vi "仪器电源管理.vi"() -> ()   [LabVIEW 2016, in "环境动力监测库.lvlib" / "电源管理库.lvlib"]
uses:
  <vilib>/Utility/miscctls.llb/LVPointTypeDef.ctl
panel:
  out "R115":i16 caption="灯带关闭时间"
  out "R114":i16 caption="灯带开启时间"
  in  "视频监控":bool
  in  "照明":bool
  in  "前门灯带":bool
  in  "侧边灯带":bool
  in  "电源控制":T1
  in  "副屏看门狗启用":u16(ring) caption="副屏看门狗启用：" items=["关闭", "打开"]
  in  "副屏看门狗设置":u16 caption="副屏看门狗设置："
  out "副屏看门狗计时":u16 caption="副屏看门狗计时："
  in  "主屏看门狗启用":u16(ring) caption="主屏看门狗启用：" items=["关闭", "打开"]
  in  "主屏看门狗设置":u16 caption="主屏看门狗设置："
  out "主屏看门狗计时":u16 caption="主屏看门狗计时："
  # "仪器电源管理"
  # "s"
  # "s"
  # "s"
  # "s"
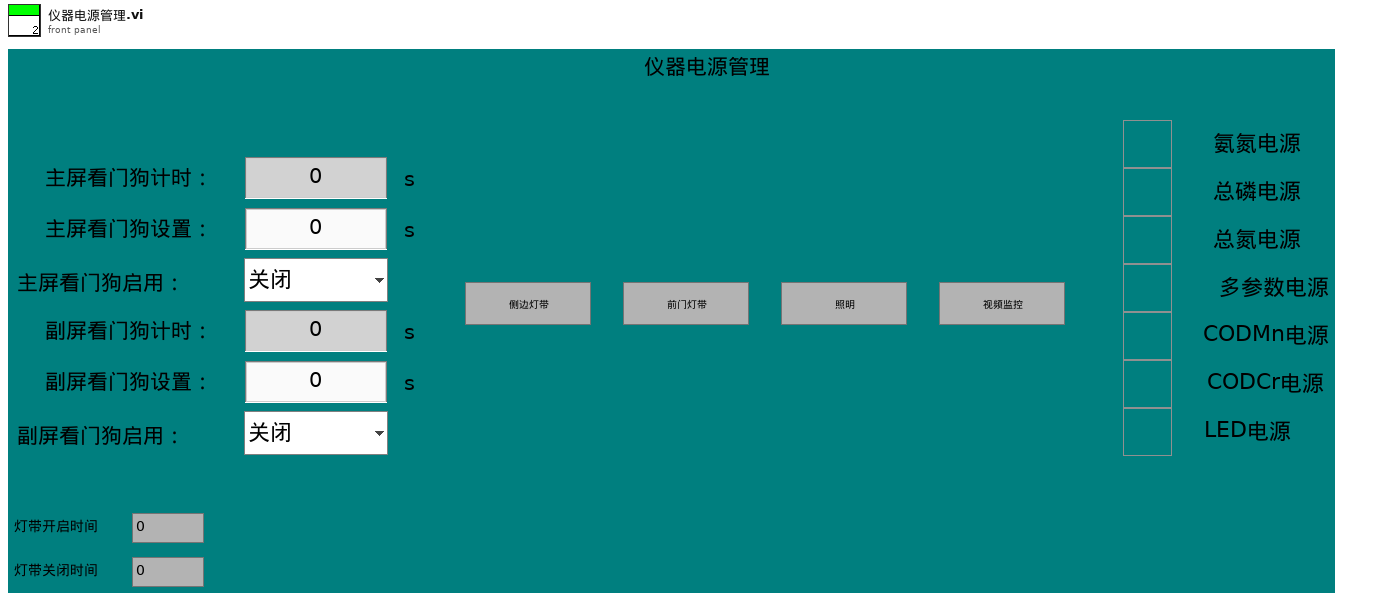
[diagram p1: front panel]
types:
  T1 = cluster{"氨氮电源":bool, "总磷电源":bool, "总氮电源":bool, "多参数电源":bool, "CODMn电源":bool, "CODCr电源":bool, "LED电源":bool}
  T2 = typedef "LVPointTypeDef.ctl" = cluster{"Horizontal":i16, "Vertical":i16}
  T3 = cluster{"R0":i16, "R1":i16, "R2":i16, "R3":i16, "R4":i16, "R5":i16, "R6":i16, "R7":i16, "R8":i16, "R9":i16, "R10":i16, "R11":i16, "R12":i16, "R13":i16, "R14":i16, "R15":i16, "R16":i16, "R17":i16, "R18":i16, "R19":i16, "R20":i16, "R21":i16, "R22":i16, "R23":i16, "R24":i16, "R25":i16, "R26":i16, "R27":i16, "R28":i16, "R29":i16, "R30":i16, "R31":i16, "R32":i16, "R33":i16, "R34":i16, "R35":i16, "R36":i16, "R37":i16, "R38":i16, "R39":i16}
  T4 = cluster{"R100":i16, "R101":i16, "R102":i16, "R103":i16, "R104":i16, "R105":i16, "R106":i16, "R107":i16, "R108":i16, "R109":i16, "R110":i16, "R111":i16, "R112":i16, "R113":i16, "R114":i16, "R115":i16, "R116":i16, "R117":i16, "R118":i16, "R119":i16, "R120":i16, "R121":i16, "R122":i16, "R123":i16}
  T5 = cluster{"命令":string, "data":cluster{"starting address":u16, "coil values":bool[]}}
  T6 = cluster{"命令":string, "数据":cluster{"starting address":u16, "holding register values":u16[]}}
  T7 = cluster{"命令":string, "数据":cluster{"starting address":u16, "holding register value":u16}}
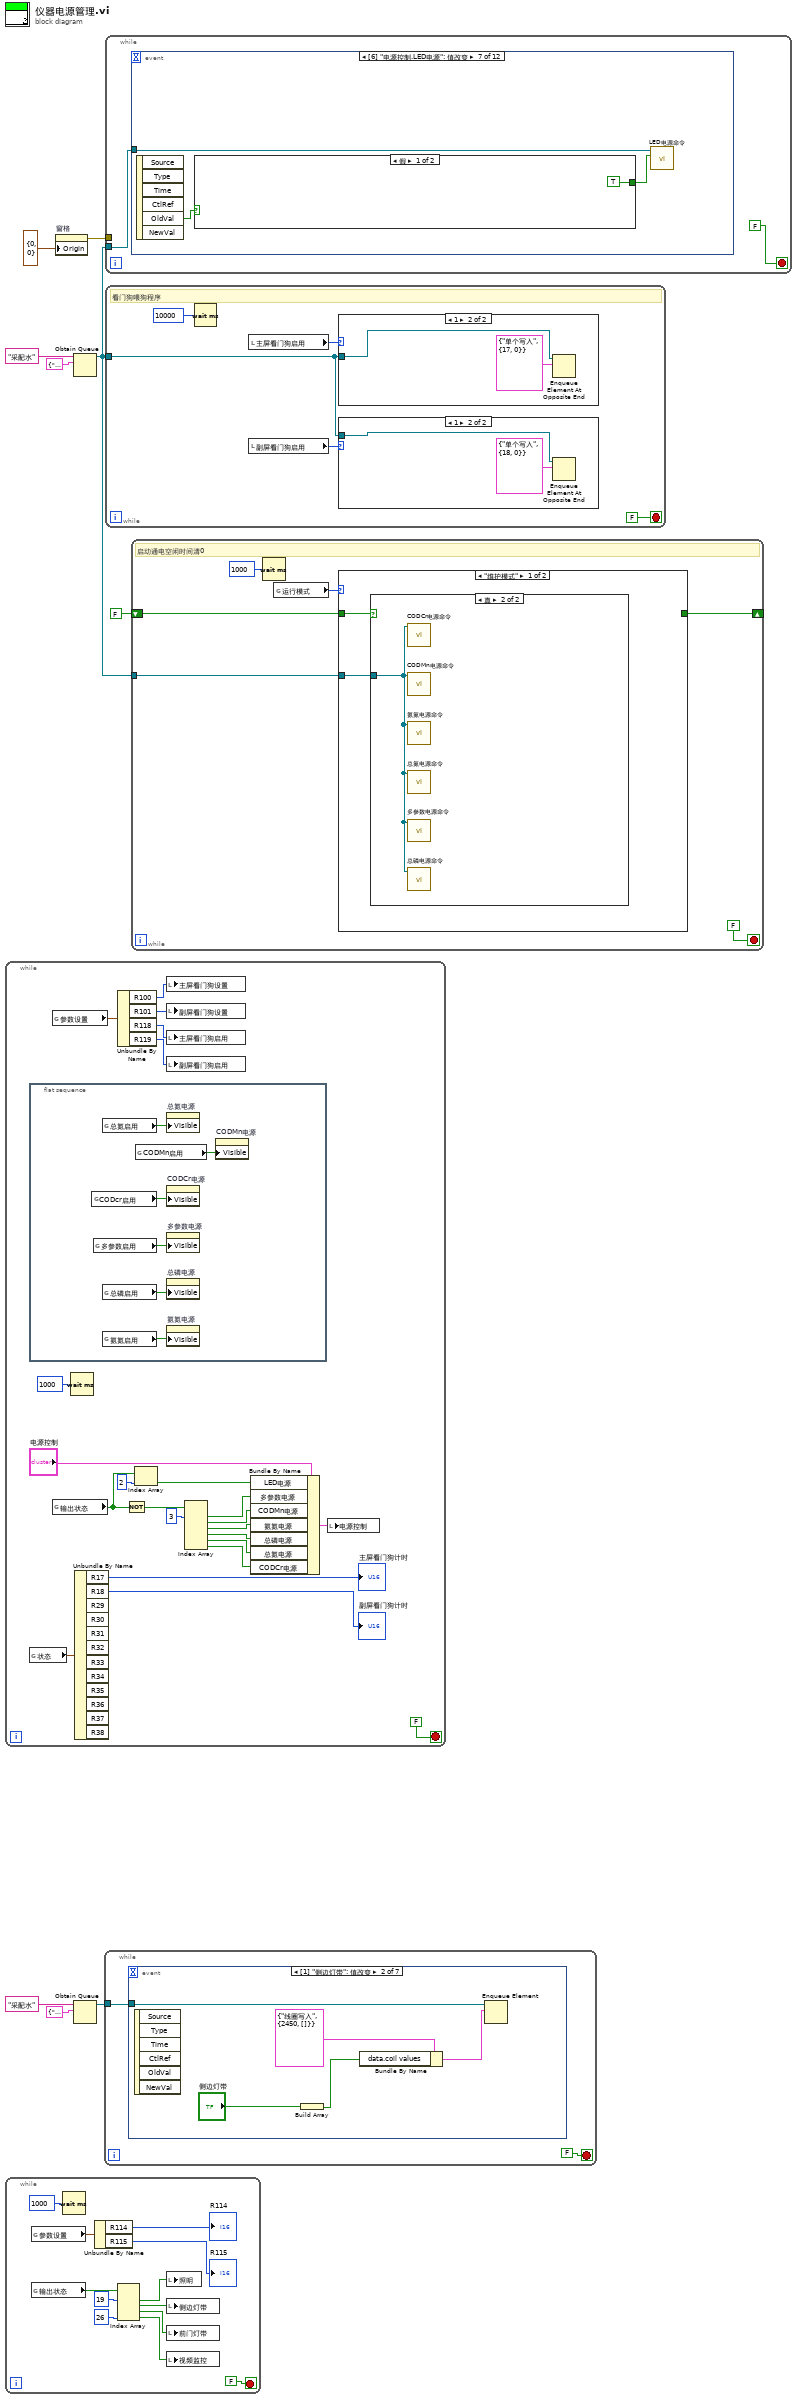
[diagram p0: block diagram]
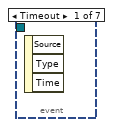
[diagram p2: hidden frame]
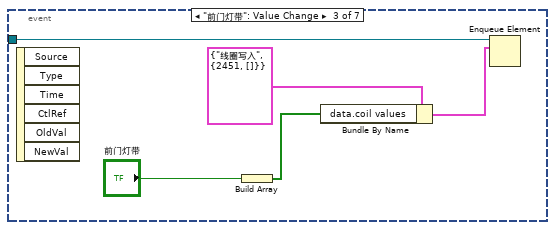
[diagram p3: hidden frame]
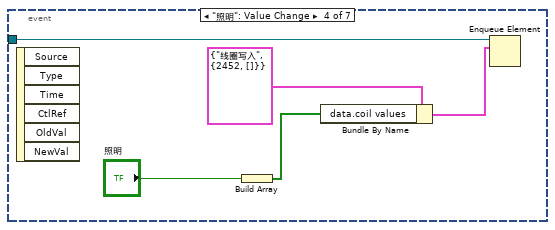
[diagram p4: hidden frame]
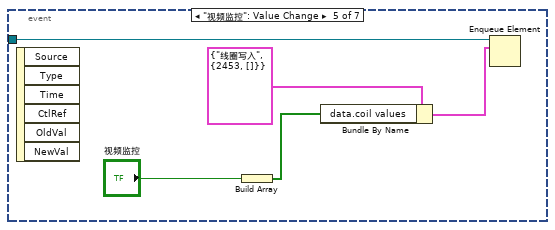
[diagram p5: hidden frame]
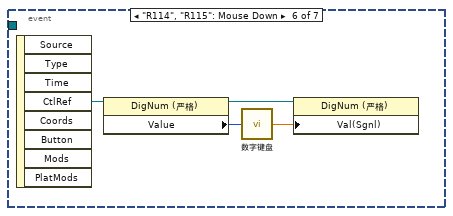
[diagram p6: hidden frame]
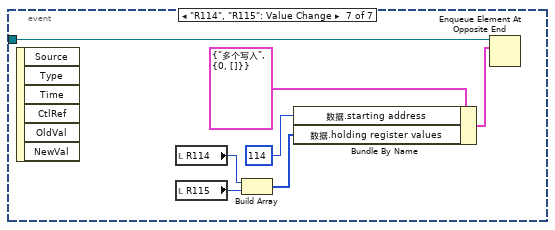
[diagram p7: hidden frame]
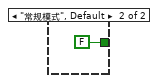
[diagram p11: hidden frame]
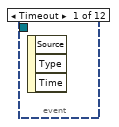
[diagram p12: hidden frame]
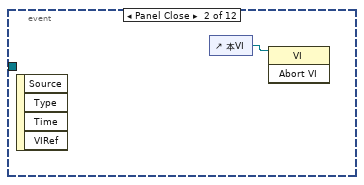
[diagram p13: hidden frame]
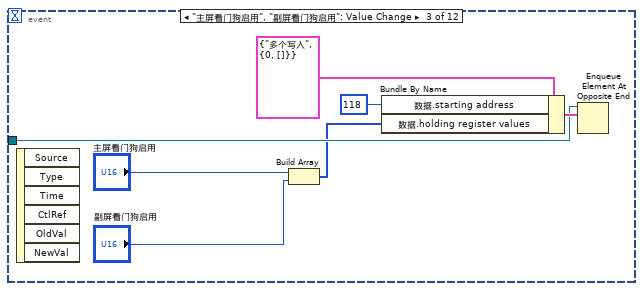
[diagram p14: hidden frame]
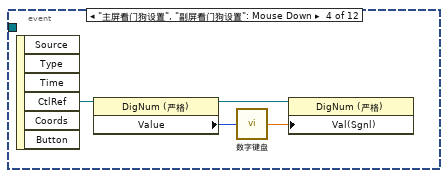
[diagram p15: hidden frame]
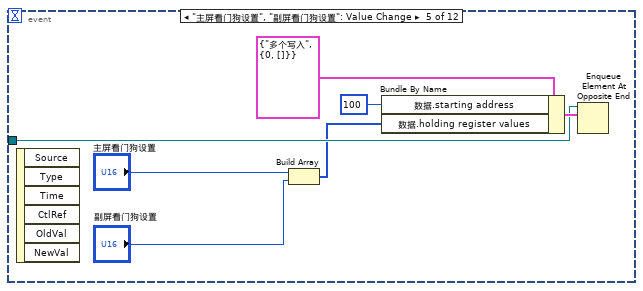
[diagram p16: hidden frame]
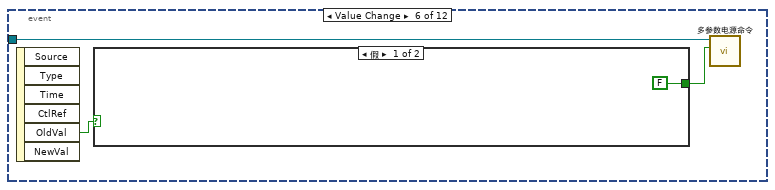
[diagram p17: hidden frame]
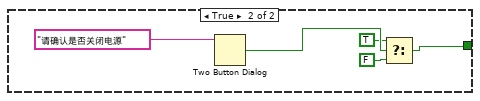
[diagram p18: hidden frame]
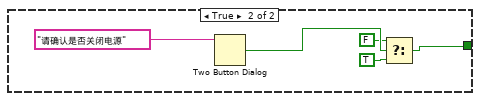
[diagram p19: hidden frame]
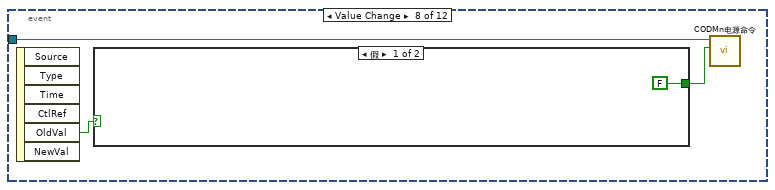
[diagram p20: hidden frame]
diagram:
  n1 = while {
    stop <- FALSE stop-if-true
    n2 = flat-sequence {
      frame #0 {
        n3 = global read "外部交互全局变量.vi" "CODcr启用"() -> (w37:bool)
        n4 = global read "外部交互全局变量.vi" "多参数启用"() -> (w33:bool)
        n5 = global read "外部交互全局变量.vi" "总氮启用"() -> (w38:bool)
        n6 = global read "外部交互全局变量.vi" "总磷启用"() -> (w36:bool)
        n7 = global read "外部交互全局变量.vi" "氨氮启用"() -> (w34:bool)
        n8 = global read "外部交互全局变量.vi" "CODMn启用"() -> (w35:bool)
        n9 = property on="总氮电源" class="Bool (严格)"("Visible"=w38) -> ()  [unwired: 2 in, 2 out]
        n10 = property on="CODCr电源" class="Bool (严格)"("Visible"=w37) -> ()  [unwired: 2 in, 2 out]
        n11 = property on="多参数电源" class="Bool (严格)"("Visible"=w33) -> ()  [unwired: 2 in, 2 out]
        n12 = property on="总磷电源" class="Bool (严格)"("Visible"=w36) -> ()  [unwired: 2 in, 2 out]
        n13 = property on="氨氮电源" class="Bool (严格)"("Visible"=w34) -> ()  [unwired: 2 in, 2 out]
        n14 = property on="CODMn电源" class="Bool (严格)"("Visible"=w35) -> ()  [unwired: 2 in, 2 out]
      }
    }
    n15 = global read "外部交互全局变量.vi" "状态"() -> (w12:T3)
    n16 = global read "外部交互全局变量.vi" "参数设置"() -> (w11:T4)
    n17 = global read "外部交互全局变量.vi" "输出状态"() -> (w10:bool[])
    n18 = Wait (ms)(milliseconds to wait=u32 1000 ("等待时间（毫秒）")) -> ()  [unwired: 1 out]
    n19 = Unbundle By Name(w12) -> ("R17"=→"主屏看门狗计时":i16, "R18"=→"副屏看门狗计时":i16)  [unwired: 10 out]
    n20 = Unbundle By Name(w11) -> ("R100"=w27:i16, "R101"=w26:i16, "R118"=w25:i16, "R119"=w24:i16)
    n21 = Not(x=w10) -> (.not. x?=w30:bool[])
    n22 = Index Array(array=w10, index=2 ("索引")) -> (element=w20:bool)
    n23 = local write "主屏看门狗设置"(w27) -> ()
    n24 = local write "副屏看门狗设置"(w26) -> ()
    n25 = local write "主屏看门狗启用"(w25) -> ()
    n26 = local write "副屏看门狗启用"(w24) -> ()
    n27 = Index Array(array=w30, index #1=3 ("索引")) -> (element #1=w19:bool, element #2=w18:bool, element #3=w17:bool, element #4=w16:bool, element #5=w15:bool, element #6=w14:bool)  [unwired: 5 in]
    n28 = Bundle By Name(cluster="电源控制", "LED电源"=w20, "多参数电源"=w19, "CODMn电源"=w18, "氨氮电源"=w17, "总磷电源"=w16, "总氮电源"=w15, "CODCr电源"=w14) -> (w13:T1)
    n29 = local write "电源控制"(w13) -> ()
  }
  n30 = while {
    stop <- FALSE stop-if-true
    n31 = global read "外部交互全局变量.vi" "参数设置"() -> (w40:T4)
    n32 = global read "外部交互全局变量.vi" "输出状态"() -> (w39:bool[])
    n33 = Wait (ms)(milliseconds to wait=u32 1000 ("等待时间（毫秒）")) -> ()  [unwired: 1 out]
    n34 = Unbundle By Name(w40) -> ("R114"=→"R114":i16, "R115"=→"R115":i16)
    n35 = Index Array(array=w39, index #1=19 ("索引"), index #4=26 ("索引")) -> (element #1=w45:bool, element #2=w44:bool, element #3=w46:bool, element #4=w43:bool)  [unwired: 2 in]
    n36 = local write "照明"(w45) -> ()
    n37 = local write "侧边灯带"(w44) -> ()
    n38 = local write "前门灯带"(w46) -> ()
    n39 = local write "视频监控"(w43) -> ()
  }
  n40 = property on="窗格" class="Pane"("Origin"=T2 {"Horizontal"=0, "Vertical"=0} ("原点")) -> (error out=w6:errorcluster)  [unwired: 2 in, 1 out]
  n41 = Obtain Queue(name (unnamed)="采配水" ("名称（未命名）"), element data type=cluster{"命令":string, "数据":variant} {"命令"="", "数据"=variant}) -> (queue out=w4:refnum<queue>)  [unwired: 3 in, 2 out]
  n42 = Obtain Queue(name (unnamed)="采配水" ("名称（未命名）"), element data type=cluster{"命令":string, "数据":variant} {"命令"="", "数据"=variant}) -> (queue out=w1:refnum<queue>)  [unwired: 3 in, 2 out]
  n43 = while {
    tunnel: w1 -> [w51]
    stop <- FALSE stop-if-true
    n44 = event shown="[1] \"侧边灯带\": 值改变" {
      selector: _ -> [_ _ _ _ _ _ _]
      dyn-events: _ -> [_ _ _ _ _ _ _]
      timeout: _ -> [_ _ _ _ _ _ _]
      tunnel: w51 -> [_ w54 w60 w65 w70 _ w77]
      event Timeout {
        n45 = event-data() -> ()  [unwired: 1 in, 3 out]
      }
      event "侧边灯带": Value Change {
        n46 = event-data() -> ()  [unwired: 1 in, 6 out]
        n47 = Build Array("侧边灯带") -> (w53:bool[])
        n48 = Bundle By Name(cluster=T5 {"命令"="线圈写入", "data"={"starting address"=2450, "coil values"=[]}} ("元素"), "data.coil values"=w53) -> (w55:T5)
        n49 = Enqueue Element(queue=w54, element=w55) -> ()  [unwired: 2 in, 3 out]
      }
      event "前门灯带": Value Change {
        n50 = event-data() -> ()  [unwired: 1 in, 6 out]
        n51 = Build Array("前门灯带") -> (w59:bool[])
        n52 = Bundle By Name(cluster=T5 {"命令"="线圈写入", "data"={"starting address"=2451, "coil values"=[]}} ("元素"), "data.coil values"=w59) -> (w61:T5)
        n53 = Enqueue Element(queue=w60, element=w61) -> ()  [unwired: 2 in, 3 out]
      }
      event "照明": Value Change {
        n54 = event-data() -> ()  [unwired: 1 in, 6 out]
        n55 = Build Array("照明") -> (w64:bool[])
        n56 = Bundle By Name(cluster=T5 {"命令"="线圈写入", "data"={"starting address"=2452, "coil values"=[]}} ("元素"), "data.coil values"=w64) -> (w66:T5)
        n57 = Enqueue Element(queue=w65, element=w66) -> ()  [unwired: 2 in, 3 out]
      }
      event "视频监控": Value Change {
        n58 = event-data() -> ()  [unwired: 1 in, 6 out]
        n59 = Build Array("视频监控") -> (w69:bool[])
        n60 = Bundle By Name(cluster=T5 {"命令"="线圈写入", "data"={"starting address"=2453, "coil values"=[]}} ("元素"), "data.coil values"=w69) -> (w71:T5)
        n61 = Enqueue Element(queue=w70, element=w71) -> ()  [unwired: 2 in, 3 out]
      }
      event "R114", "R115": Mouse Down {
        n62 = event-data() -> ("CtlRef"=w76:refnum<vi>)  [unwired: 1 in, 7 out]
        n63 = property class="DigNum (严格)"(reference=w76) -> (reference out=w75:refnum<vi>, "Value"=w74:i16)  [unwired: 1 in, 1 out]
        n64 = call "数字键盘.vi"("OldNumber"=w74) -> ("NewNumber"=w73:sgl)
        n65 = property class="DigNum (严格)"(reference=w75, "Val(Sgnl)"=w73) -> ()  [unwired: 1 in, 2 out]
      }
      event "R114", "R115": Value Change {
        n66 = event-data() -> ()  [unwired: 1 in, 6 out]
        n67 = local read "R114"() -> (w82:i16)
        n68 = local read "R115"() -> (w83:i16)
        n69 = Build Array(w82, w83) -> (w78:i16[])
        n70 = Bundle By Name(cluster=T6 {"命令"="多个写入", "数据"={"starting address"=0, "holding register values"=[]}} ("元素"), "数据.starting address"=u16 114, "数据.holding register values"=w78) -> (w79:T6)
        n71 = Enqueue Element At Opposite End(queue=w77, element=w79) -> ()  [unwired: 2 in, 3 out]
      }
    }
  }
  n72 = while {
    tunnel: w4 -> [w85]
    tunnel: w6 -> [_]
    stop <- FALSE stop-if-true
    n73 = event shown="[6] \"电源控制.LED电源\": 值改变" {
      selector: _ -> [_ _ _ _ _ _ _ _ _ _ _ _]
      dyn-events: _ -> [_ _ _ _ _ _ _ _ _ _ _ _]
      timeout: _ -> [_ _ _ _ _ _ _ _ _ _ _ _]
      tunnel: w85 -> [_ _ w90 _ w101 w107 w115 w125 w134 w143 w152 w161]
      event Timeout {
        n74 = event-data() -> ()  [unwired: 1 in, 3 out]
      }
      event Panel Close {
        n75 = event-data() -> ()  [unwired: 1 in, 4 out]
        n76 = control-ref of="本VI"() -> (w86:refnum<vi>)
        n77 = invoke class="VI" method="Abort VI"(reference=w86) -> ()  [unwired: 2 in, 3 out]
      }
      event "主屏看门狗启用", "副屏看门狗启用": Value Change {
        n78 = event-data() -> ()  [unwired: 1 in, 6 out]
        n79 = Build Array("主屏看门狗启用", "副屏看门狗启用") -> (w87:u16[])
        n80 = Bundle By Name(cluster=T6 {"命令"="多个写入", "数据"={"starting address"=0, "holding register values"=[]}} ("元素"), "数据.starting address"=u16 118, "数据.holding register values"=w87) -> (w91:T6)
        n81 = Enqueue Element At Opposite End(queue=w90, element=w91) -> ()  [unwired: 2 in, 3 out]
      }
      event "主屏看门狗设置", "副屏看门狗设置": Mouse Down {
        n82 = event-data() -> ("CtlRef"=w94:refnum<vi>)  [unwired: 1 in, 5 out]
        n83 = property class="DigNum (严格)"(reference=w94) -> (reference out=w96:refnum<vi>, "Value"=w97:u16)  [unwired: 1 in, 1 out]
        n84 = call "数字键盘.vi"("OldNumber"=w97) -> ("NewNumber"=w95:sgl)
        n85 = property class="DigNum (严格)"(reference=w96, "Val(Sgnl)"=w95) -> ()  [unwired: 1 in, 2 out]
      }
      event "主屏看门狗设置", "副屏看门狗设置": Value Change {
        n86 = event-data() -> ()  [unwired: 1 in, 6 out]
        n87 = Build Array("主屏看门狗设置", "副屏看门狗设置") -> (w98:u16[])
        n88 = Bundle By Name(cluster=T6 {"命令"="多个写入", "数据"={"starting address"=0, "holding register values"=[]}} ("元素"), "数据.starting address"=u16 100, "数据.holding register values"=w98) -> (w102:T6)
        n89 = Enqueue Element At Opposite End(queue=w101, element=w102) -> ()  [unwired: 2 in, 3 out]
      }
      event "电源控制.多参数电源": Value Change {
        n90 = event-data() -> ("OldVal"=w106:bool)  [unwired: 1 in, 5 out]
        n91 = case shown="假" w106 {
          tunnel: [FALSE ("T button?") w109] -> w105
          frame False {
          }
          frame True {
            n92 = Two Button Dialog(message="请确认是否关闭电源" ("消息")) -> (T button?=w112:bool)  [unwired: 2 in]
            n93 = Select(t=TRUE, s=w112, f=FALSE ("T button?")) -> (s? t:f=w109:bool)
          }
        }
        n94 = call "多参数电源命令.vi"("通电/断电"=w105, "队列"=w107) -> ()  [unwired: 9 in, 1 out]
      }
      event "电源控制.LED电源": Value Change {
        n95 = event-data() -> ("OldVal"=w116:bool)  [unwired: 1 in, 5 out]
        n96 = case shown="假" w116 {
          tunnel: [TRUE ("T button?") w118] -> w114
          frame False {
          }
          frame True {
            n97 = Two Button Dialog(message="请确认是否关闭电源" ("消息")) -> (T button?=w121:bool)  [unwired: 2 in]
            n98 = Select(t=FALSE, s=w121, f=TRUE ("T button?")) -> (s? t:f=w118:bool)
          }
        }
        n99 = call "LED电源命令.vi"("通电/断电"=w114, "队列"=w115) -> ()  [unwired: 9 in, 1 out]
      }
      event "电源控制.CODMn电源": Value Change {
        n100 = event-data() -> ("OldVal"=w124:bool)  [unwired: 1 in, 5 out]
        n101 = case shown="假" w124 {
          tunnel: [FALSE ("T button?") w127] -> w123
          frame False {
          }
          frame True {
            n102 = Two Button Dialog(message="请确认是否关闭电源" ("消息")) -> (T button?=w130:bool)  [unwired: 2 in]
            n103 = Select(t=TRUE, s=w130, f=FALSE ("T button?")) -> (s? t:f=w127:bool)
          }
        }
        n104 = call "CODMn电源命令.vi"("通电/断电"=w123, "队列"=w125) -> ()  [unwired: 9 in, 1 out]
      }
      event "电源控制.氨氮电源": Value Change {
        n105 = event-data() -> ("OldVal"=w133:bool)  [unwired: 1 in, 5 out]
        n106 = case shown="假" w133 {
          tunnel: [FALSE ("T button?") w136] -> w132
          frame False {
          }
          frame True {
            n107 = Two Button Dialog(message="请确认是否关闭电源" ("消息")) -> (T button?=w139:bool)  [unwired: 2 in]
            n108 = Select(t=TRUE, s=w139, f=FALSE ("T button?")) -> (s? t:f=w136:bool)
          }
        }
        n109 = call "氨氮电源命令.vi"("通电/断电"=w132, "队列"=w134) -> ()  [unwired: 9 in, 1 out]
      }
      event "电源控制.总磷电源": Value Change {
        n110 = event-data() -> ("OldVal"=w142:bool)  [unwired: 1 in, 5 out]
        n111 = case shown="假" w142 {
          tunnel: [FALSE ("T button?") w145] -> w141
          frame False {
          }
          frame True {
            n112 = Two Button Dialog(message="请确认是否关闭电源" ("消息")) -> (T button?=w148:bool)  [unwired: 2 in]
            n113 = Select(t=TRUE, s=w148, f=FALSE ("T button?")) -> (s? t:f=w145:bool)
          }
        }
        n114 = call "总磷电源命令.vi"("通电/断电"=w141, "队列"=w143) -> ()  [unwired: 9 in, 1 out]
      }
      event "电源控制.CODCr电源": Value Change {
        n115 = event-data() -> ("OldVal"=w151:bool)  [unwired: 1 in, 5 out]
        n116 = case shown="假" w151 {
          tunnel: [FALSE ("T button?") w154] -> w150
          frame False {
          }
          frame True {
            n117 = Two Button Dialog(message="请确认是否关闭电源" ("消息")) -> (T button?=w157:bool)  [unwired: 2 in]
            n118 = Select(t=TRUE, s=w157, f=FALSE ("T button?")) -> (s? t:f=w154:bool)
          }
        }
        n119 = call "CODCr电源命令.vi"("通电/断电"=w150, "队列"=w152) -> ()  [unwired: 9 in, 1 out]
      }
      event "电源控制.总氮电源": Value Change {
        n120 = event-data() -> ("OldVal"=w159:bool)  [unwired: 1 in, 5 out]
        n121 = case shown="假" w159 {
          tunnel: [FALSE ("T button?") w163] -> w160
          frame False {
          }
          frame True {
            n122 = Two Button Dialog(message="请确认是否关闭电源" ("消息")) -> (T button?=w166:bool)  [unwired: 2 in]
            n123 = Select(t=TRUE, s=w166, f=FALSE ("T button?")) -> (s? t:f=w163:bool)
          }
        }
        n124 = call "总氮电源命令.vi"("通电/断电"=w160, "队列"=w161) -> ()  [unwired: 9 in, 1 out]
      }
    }
  }
  n125 = while {
    tunnel: w4 -> [w172]
    stop <- FALSE stop-if-true
    # "看门狗喂狗程序"
    n126 = Wait (ms)(milliseconds to wait=u32 10000 ("等待时间（毫秒）")) -> ()  [unwired: 1 out]
    n127 = local read "主屏看门狗启用"() -> (w171:u16)
    n128 = local read "副屏看门狗启用"() -> (w170:u16)
    n129 = case shown="1" w171 {
      tunnel: w172 -> [_ w175]
      frame 0, Default {
      }
      frame 1 {
        n130 = Enqueue Element At Opposite End(queue=w175, element=T7 {"命令"="单个写入", "数据"={"starting address"=17, "holding register value"=0}} ("元素")) -> ()  [unwired: 2 in, 3 out]
      }
    }
    n131 = case shown="1" w170 {
      tunnel: w172 -> [_ w173]
      frame 0, Default {
      }
      frame 1 {
        n132 = Enqueue Element At Opposite End(queue=w173, element=T7 {"命令"="单个写入", "数据"={"starting address"=18, "holding register value"=0}} ("元素")) -> ()  [unwired: 2 in, 3 out]
      }
    }
  }
  n133 = while {
    tunnel: w4 -> [w180]
    shift-right: [w178] -> _
    shift-left: FALSE -> [w179]
    stop <- FALSE stop-if-true
    # "启动通电空闲时间清0"
    n134 = Wait (ms)(milliseconds to wait=u32 1000 ("等待时间（毫秒）")) -> ()  [unwired: 1 out]
    n135 = global read "外部交互全局变量.vi" "运行模式"() -> (w177:enum16{"维护模式", "常规模式", "应急模式", "质控模式"})
    n136 = case shown="\"维护模式\"" w177 {
      tunnel: w180 -> [w184 _]
      tunnel: w179 -> [w183 _]
      tunnel: [_ FALSE] -> w178
      frame "维护模式" {
        n137 = case shown="真" w183 {
          tunnel: w184 -> [_ w185]
          frame False {
          }
          frame True {
            n138 = call "CODCr电源命令.vi"("队列"=w185) -> ()  [unwired: 10 in, 1 out]
            n139 = call "CODMn电源命令.vi"("队列"=w185) -> ()  [unwired: 10 in, 1 out]
            n140 = call "氨氮电源命令.vi"("队列"=w185) -> ()  [unwired: 10 in, 1 out]
            n141 = call "总氮电源命令.vi"("队列"=w185) -> ()  [unwired: 10 in, 1 out]
            n142 = call "多参数电源命令.vi"("队列"=w185) -> ()  [unwired: 10 in, 1 out]
            n143 = call "总磷电源命令.vi"("队列"=w185) -> ()  [unwired: 10 in, 1 out]
          }
        }
      }
      frame "常规模式", Default {
      }
    }
  }
